vi "getROIfromCoords.vi"(0 "x1":i32, 1 "y1":i32, 2 "x2":i32, 3 "y2":i32, 4 "type":u32) -> (5 "ROI":T1)   [LabVIEW 2015]
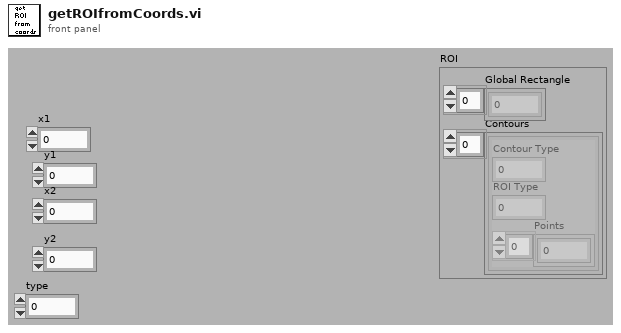
[diagram p1: front panel]
types:
  T1 = cluster{"Global Rectangle":i32[], "Contours":cluster{"Contour Type":u32, "ROI Type":u32, "Points":i32[]}[]}
  T2 = cluster{i32[], cluster{u32, "type":u32, i32[]}[]}
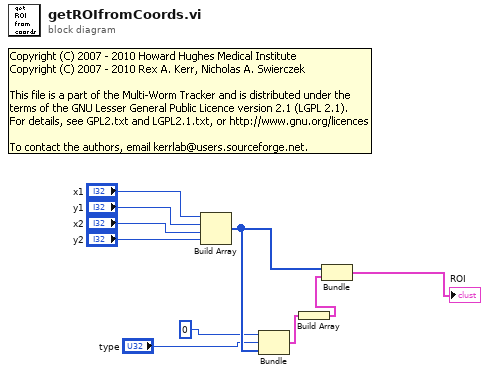
[diagram p0: block diagram]
diagram:
  n1 = Build Array("x1", "y1", "x2", "y2") -> (w6:i32[])
  n2 = Bundle(u32 0, "type"="type", w6) -> (w3:cluster{u32, "type":u32, i32[]})  [unwired: 1 in]
  n3 = Build Array(w3) -> (w2:cluster{u32, "type":u32, i32[]}[])
  n4 = Bundle(w6, w2) -> (→"ROI":T2)  [unwired: 1 in]
